vi "PXI_Host_Bool_Read_NewMethod_Benchmark.vi"() -> ()   [LabVIEW 2018]
uses:
  <vilib>/Platform/TimedLoop/XDataNode/timing_clust.ctl
  <vilib>/Platform/TimedLoop/XDataNode/nitl_modes.ctl
  <vilib>/Platform/TimedLoop/XDataNode/wakeup.ctl
  cRIO RT/FPGA Bitfile Register Operations/Scalar IO Operations/Read Methods/Read Data Register/Instances/Read Boolean.vi
  cRIO RT/FPGA Bitfile Register Operations/Scalar IO Operations/Utilities/Find Register Offset.vi
  cRIO RT/FPGA Bitfile Register Operations/Scalar IO Operations/SubVIs/Check Register Data Store.vi
  cRIO RT/FPGA Bitfile Register Operations/Scalar IO Operations/Error Handling/Error 6001.vi
  cRIO RT/FPGA Bitfile Register Operations/Scalar IO Operations/Error Handling/Error 6000.vi
  cRIO RT/FPGA Bitfile Register Operations/Scalar IO Operations/Error Handling/Error 6002.vi
  cRIO RT/FPGA Bitfile Register Operations/Scalar IO Operations/Error Handling/Error 6003.vi
  <vilib>/FPGAPlugInAG/Dynamic/niLvFpga_Close_Dynamic.vi
  <vilib>/platform/TimedLoop/XDataNode/XDataNode.xnode
  <vilib>/rvi/interface/nirviCloseFPGA/nirviCloseFPGA.xnode
  cRIO RT/FPGA Bitfile Register Operations/Scalar IO Operations/FPGA Register IO.lvlib
  <vilib>/Platform/TimedLoop/XDataNode/XDNodeRunTimeDep.lvlib
panel:
  out "Waveform Graph":dbl[](graph)
  out "Standard Dev":dbl
  out "Execution time (s)":dbl
  out "Maximum(s)":dbl
  out "Value out":bool
  out "error out":errorcluster
  # "Recorded time"
  # "3.37551E-5"
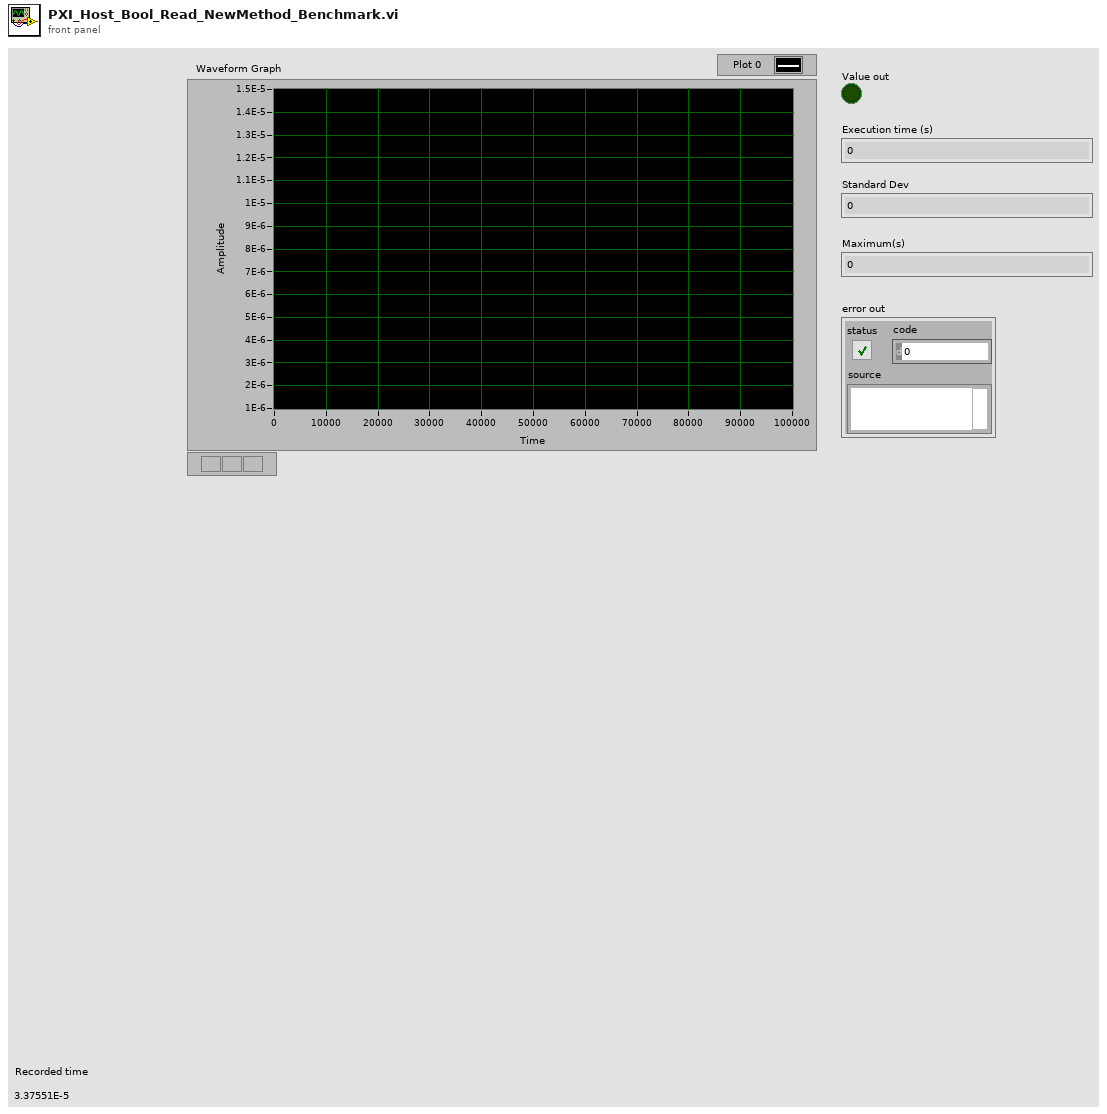
[diagram p1: front panel]
types:
  T1 = typedef "XDNodeRunTimeDep.lvlib/timing_clust.ctl" = cluster{"Expected End [f-1]":u64, "Actual End [f-1]":u64, "Finished Late? [f-1]":bool, "Expected End [i-1]":u64, "Actual End [i-1]":u64, "Finished Late? [i-1]":bool, "Expected Start [i]":u64, "Actual Start [i]":u64, "Expected Start [f]":u64, "Actual Start [f]":u64, "Source Name":string, "Structure Name":string, "Period":i64, "Deadline":i64, "Offset":i64, "Start":i64, "Priority":i32, "Timeout":i32, "Mode":T2, "Wakeup Reason":T3, "Error":errorcluster, "Source Type":string, "Secondary Source Type":string, "Global End Time":u64, "Global Start Time":u64, "Frame Duration":u64, "Iteration Duration":u64, "Assigned CPU":i32, "I/O Scan Engine Mode":u32}
  T2 = typedef "XDNodeRunTimeDep.lvlib/nitl_modes.ctl" = enum32{"No Change", "Process missed periods, maintain original phase", "Discard missed periods, maintain original phase", "Process missed periods, ignore original phase", "Discard missed periods, ignore original phase"}
  T3 = typedef "XDNodeRunTimeDep.lvlib/wakeup.ctl" = enum32{"Normal", "Aborted", "Asynchronous wakeup", "Timing source error", "Timed loop error", "Timeout"}
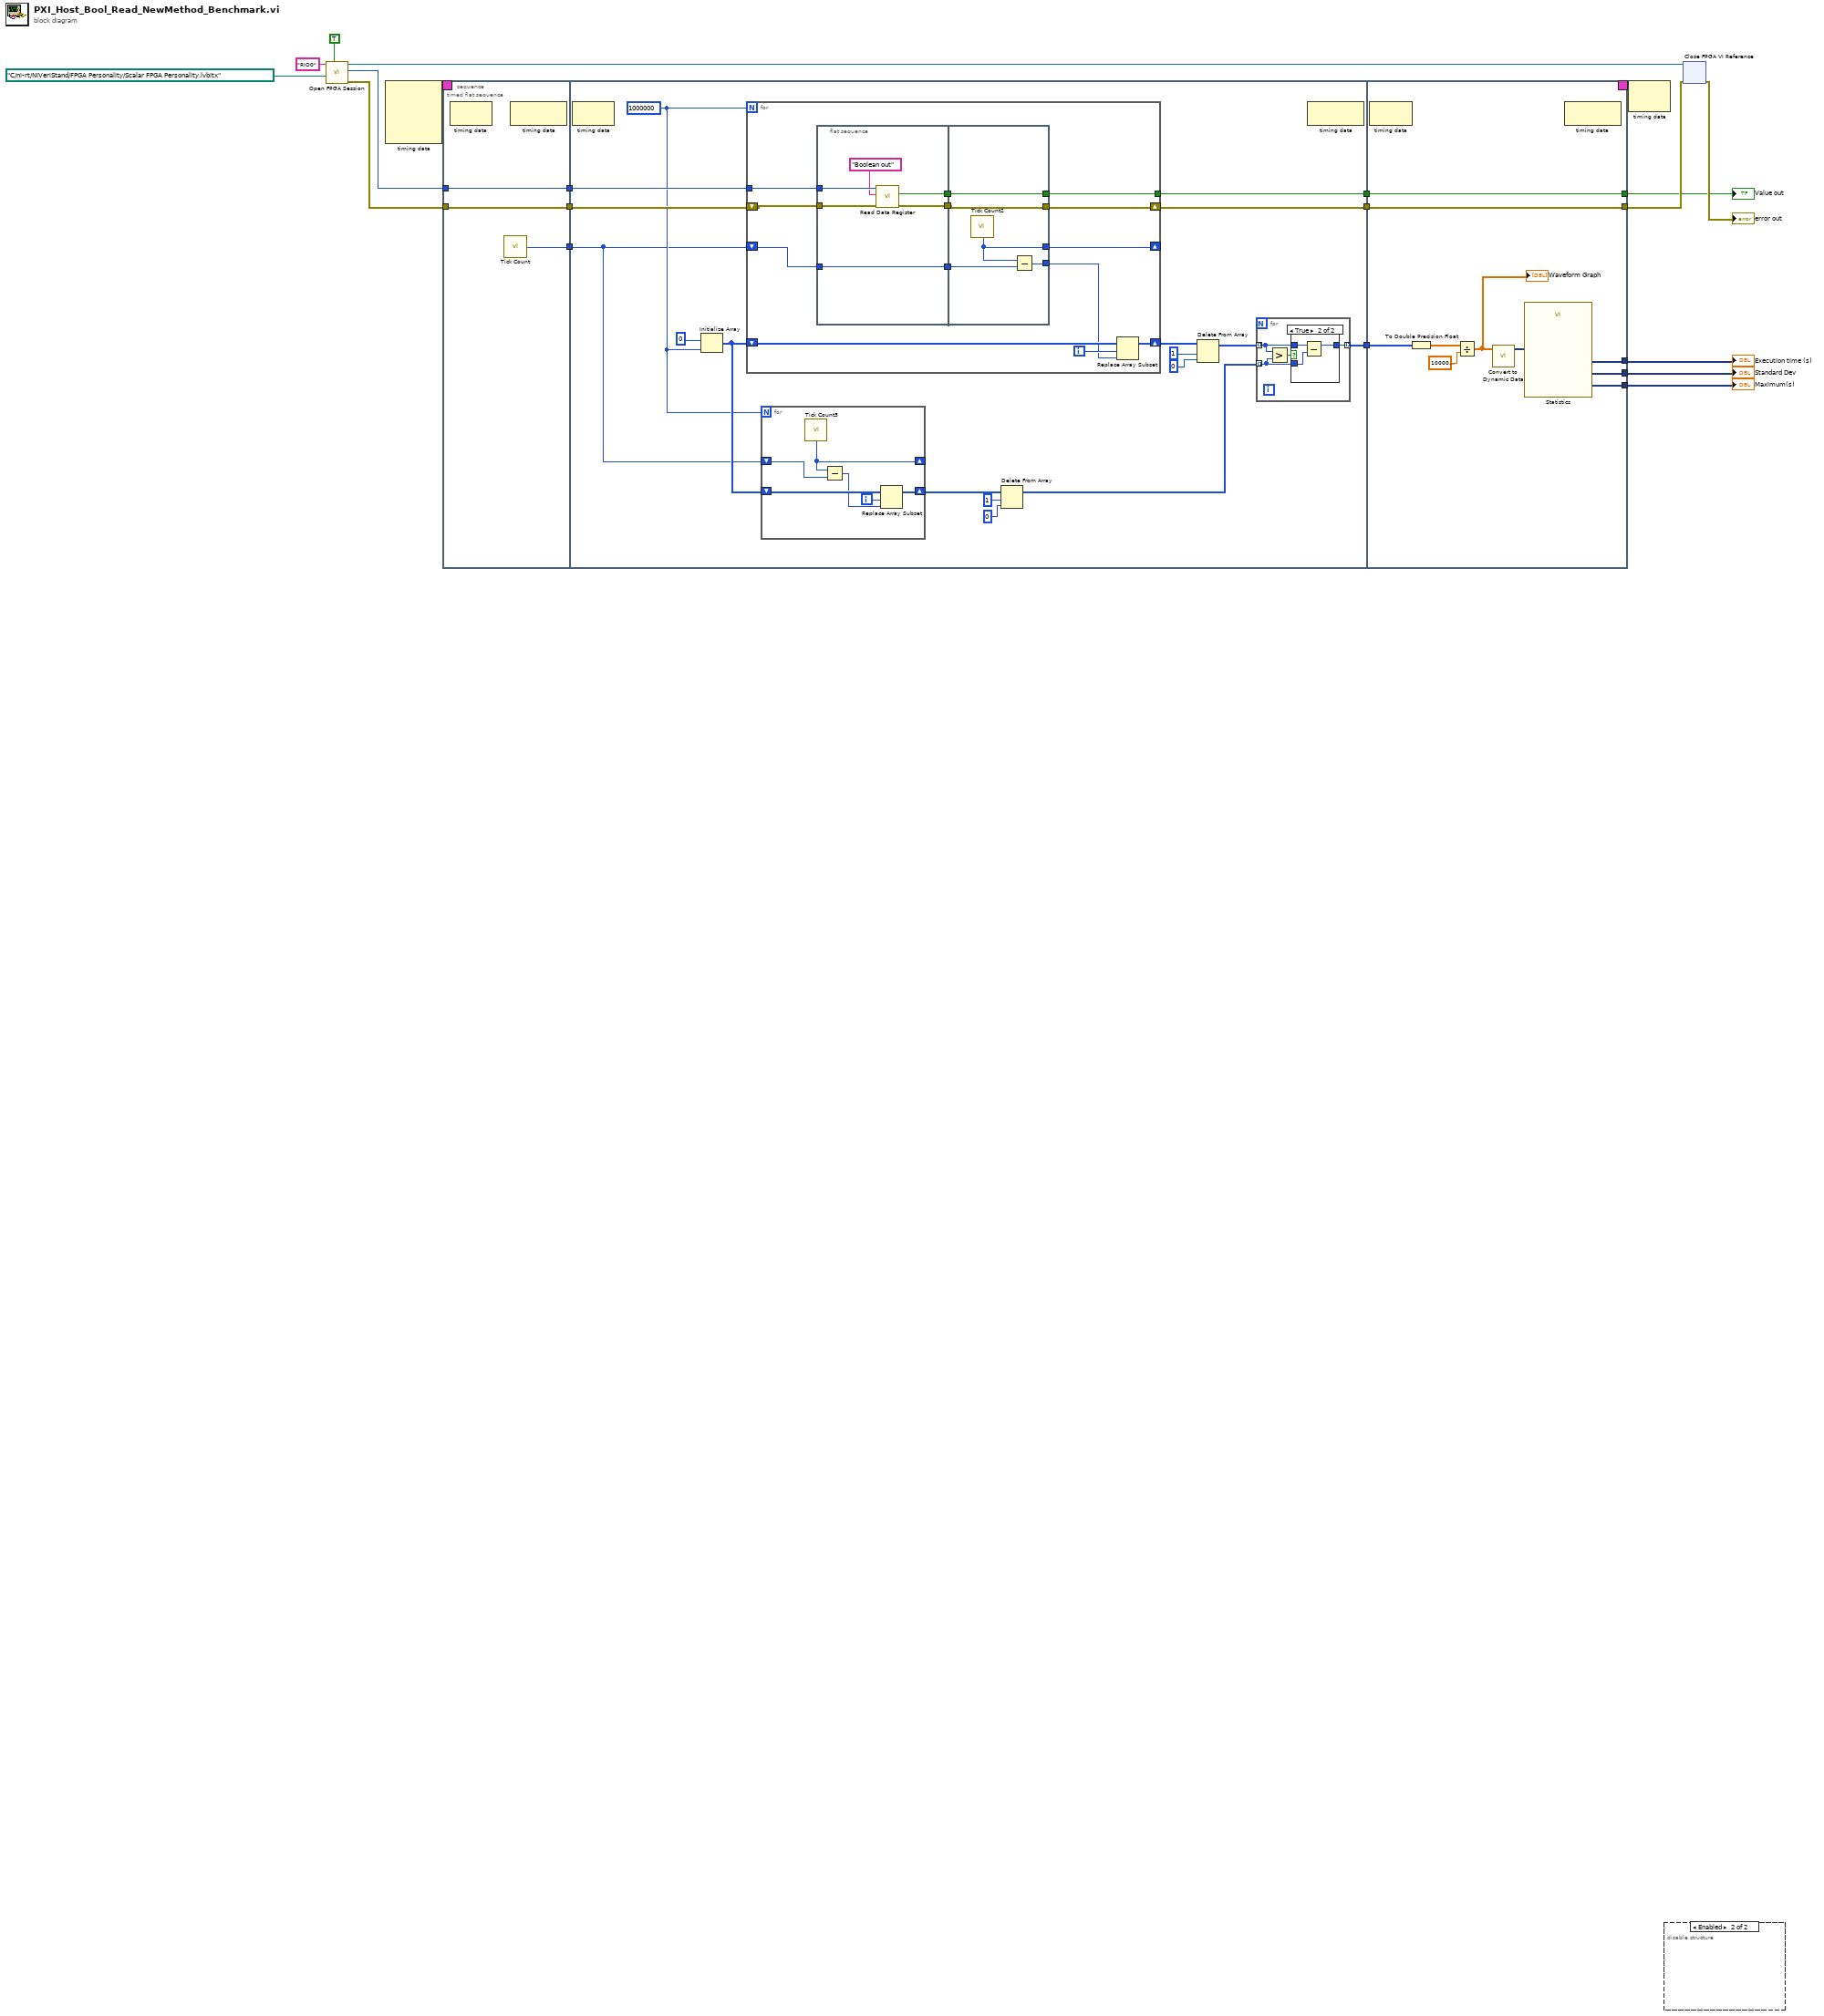
[diagram p0: block diagram]
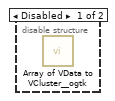
[diagram p3: hidden frame]
diagram:
  n1 = call "Open FPGA Session.vi"("run when loaded (T)"=TRUE, "bitfile path"=path "C:/ni-rt/NIVeriStand/FPGA Personality/Scalar FPGA Personality.lvbitx", "device address"="RIO0") -> ("error out"=w10:errorcluster, "session out"=w14:u32, "bitfile reference out"=w9:refnum<k20>)  [unwired: 6 in]
  n2 = node-c288() -> (w5:T1)  [unwired: 4 in]
  n3 = timed-sequence {
    timing: w5 -> [_]
    timing-out: [_] -> w4
    tunnel: w14 -> [w27]
    tunnel: w10 -> [w26]
    tunnel: [w25] -> w8
    tunnel: [w24] -> w6
    tunnel: [w17] -> w3
    tunnel: [w16] -> w2
    tunnel: [w15] -> w1
    n4 = timed-flat-sequence {
      tunnel: w26 -> [w29]
      tunnel: w27 -> [w30]
      tunnel: [w30] -> w23
      tunnel: [w29] -> w22
      tunnel: [w28] -> w21
      tunnel: w23 -> [w49]
      tunnel: w22 -> [w48]
      tunnel: w21 -> [w33]
      tunnel: [w47] -> w20
      tunnel: [w46] -> w19
      tunnel: [w35] -> w18
      tunnel: [w98] -> w24
      tunnel: [w99] -> w25
      tunnel: w20 -> [w99]
      tunnel: w19 -> [w98]
      tunnel: w18 -> [w94]
      tunnel: [w93] -> w17
      tunnel: [w92] -> w16
      tunnel: [w91] -> w15
      frame #0 {
        n5 = node-c288() -> ()  [unwired: 1 in, 1 out]
        n6 = call "Tick Count"() -> ("Tick Count(Ticks)"=w28:u32)
        n7 = node-c288() -> ()  [unwired: 1 in, 1 out]
      }
      frame #1 {
        w34 = 1000000
        n8 = node-c288() -> ()  [unwired: 1 in, 1 out]
        n9 = Initialize Array(u32 0 ("Tick Count(uSec)"), w34) -> (w44:u32[])
        n10 = for {
          N: w34 -> [_]
          tunnel: w49 -> [w69]
          tunnel: [w66] -> w46
          shift-right: [w67] -> w47
          shift-left: w48 -> [w68]
          shift-right: [w63] -> w38
          shift-left: w44 -> [w65]
          shift-right: [w60] -> _
          shift-left: w33 -> [w62]
          i -> [w64]
          n11 = flat-sequence {
            tunnel: [w78] -> w72
            tunnel: [w75] -> w71
            tunnel: [w74] -> w70
            tunnel: w62 -> [w78]
            tunnel: w69 -> [w77]
            tunnel: w68 -> [w76]
            tunnel: w72 -> [w83]
            tunnel: [w82] -> w61
            tunnel: w71 -> [w81]
            tunnel: [w81] -> w67
            tunnel: w70 -> [w80]
            tunnel: [w80] -> w66
            tunnel: [w79] -> w60
            frame #0 {
              n12 = call-poly "Read Data Register.vi"("error in"=w76, "register name"="Boolean out", "session in"=w77) -> ("error out"=w75:errorcluster, "value out"=w74:bool)  [unwired: 6 in, 1 out]
            }
            frame #1 {
              n13 = call "Tick Count2"() -> ("Tick Count(Ticks)"=w79:u32)
              n14 = Subtract(x=w79, y=w83) -> (x-y=w82:u32)
            }
          }
          n15 = Replace Array Subset(array=w65, new element=w61, index=w64) -> (w63:u32[])
        }
        n16 = for {
          N: w34 -> [_]
          shift-right: [w84] -> w41
          shift-left: w44 -> [w87]
          shift-right: [w89] -> _
          shift-left: w33 -> [w88]
          i -> [w85]
          n17 = call "Tick Count3"() -> ("Tick Count(Ticks)"=w89:u32)
          n18 = Subtract(x=w89, y=w88) -> (x-y=w86:u32)
          n19 = Replace Array Subset(array=w87, new element=w86, index=w85) -> (w84:u32[])
        }
        n20 = Delete From Array(array=w41, length=1, index=0) -> (array with subset deleted=w36:u32[])  [unwired: 1 out]
        n21 = Delete From Array(array=w38, length=1, index=0) -> (array with subset deleted=w37:u32[])  [unwired: 1 out]
        n22 = for {
          tunnel: [w55] -> w35 mode=indexing
          tunnel: w37 -> [w54] mode=indexing
          tunnel: w36 -> [w53] mode=indexing
          n23 = Greater?(x=w54, y=w53) -> (0:w52:bool)
          n24 = case shown="True" w52 {
            tunnel: w54 -> [w56 w59]
            tunnel: w53 -> [_ w58]
            tunnel: [w56 w57] -> w55
            frame False {
            }
            frame True {
              n25 = Subtract(x=w59, y=w58) -> (x-y=w57:u32)
            }
          }
        }
        n26 = node-c288() -> ()  [unwired: 1 in, 1 out]
      }
      frame #2 {
        n27 = node-c288() -> ()  [unwired: 1 in, 1 out]
        n28 = To Double Precision Float(number=w94) -> (double precision float=w97:dbl[])
        n29 = Divide(x=w97, y=1000000000.0) -> (x/y=w90:dbl[])
        "Waveform Graph" <- w90
        n30 = call "Convert to Dynamic Data"("Array"=w90) -> ("Dynamic Data Type"=w95:dynamicdata)  [unwired: 3 in]
        n31 = call "Statistics"("Signals"=w95) -> ("Standard Dev"=w92:dynamicdata, "Arithmetic Mean"=w93:dynamicdata, "Maximum"=w91:dynamicdata)  [unwired: 23 in, 1 out]
        n32 = node-c288() -> ()  [unwired: 1 in, 1 out]
      }
    }
  }
  "Value out" <- w6
  "Maximum(s)" <- w1
  "Execution time (s)" <- w3
  "Standard Dev" <- w2
  n33 = node-c288(w4) -> ()  [unwired: 1 out]
  n34 = disable-structure shown="Enabled" {
    frame Disabled {
      n35 = call <userlib>:"Array of VData to VCluster__ogtk.vi"() -> ()  [unwired: 10 in, 2 out]
    }
    frame Enabled {
    }
  }
  n36 = xnode "Close FPGA VI Reference"("FPGA VI Reference In"=w9, "error in"=w8) -> ("error out"=→"error out":errorcluster)
